vi "read.vi"(8 "error in (no error)":errorcluster, 11 "ValuePass in":refnum<class "RPCVariable.lvclass">) -> (0 "error out":errorcluster, 1 "Numeric":dbl, 2 "String":string, 3 "ValuePass out":refnum<class "RPCVariable.lvclass">)   [LabVIEW 2011, in "mbed_LVLibrary.lvlib" / "RPCVariable.lvclass"]
doc: "This VI will read the value of an RPCVariable on mbed. If the value is numeric it will be avalible on the numeric pin in number format, otherwise if it cannot be formatted to a number it will only be avalible as a string. When using this you need to be aware of the type of the variable attached on mbed."
uses:
  RPCVariable.lvclass
  RPCVariable.lvclass/RPCVariable.ctl
  Transport Mechanisms/mbed/mbed.lvclass
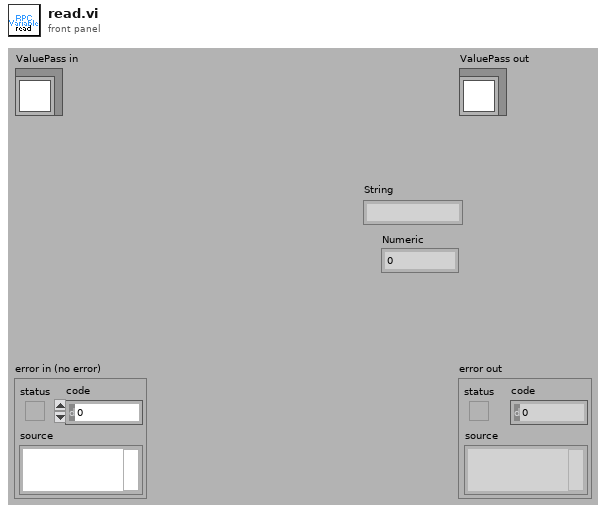
[diagram p1: front panel]
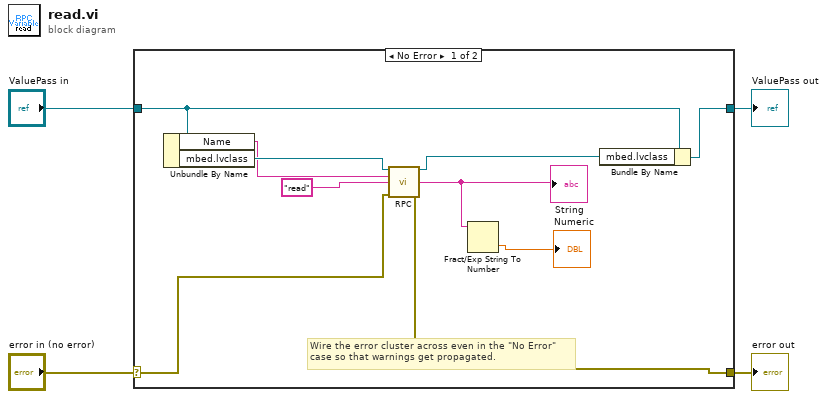
[diagram p0: block diagram]
diagram:
  n1 = case shown="No Error" "error in (no error)" {
    selector: "error in (no error)" -> [w8 w16]
    tunnel: [w7 w16] -> w3
    tunnel: [w13 w15] -> w1
    tunnel: "ValuePass in" -> [w14 w15]
    frame No Error {
      # "Wire the error cluster across even in the \"No Error\"\ncase so that warnings get propagated."
      n2 = Unbundle By Name(w14) -> ("Name"=w11:string, "mbed.lvclass"=w12:refnum<class "mbed.lvclass">)
      n3 = call-dynamic "RPC.vi"("mbed in"=w12, "Name"=w11, "method"="read", "error in (no error)"=w8) -> ("mbed out"=w10:refnum<class "mbed.lvclass">, "RPC Result"=w6:string, "error out"=w7:errorcluster)  [unwired: 9 in]
      "String" <- w6
      n4 = Fract/Exp String To Number(string=w6) -> (number=→"Numeric":dbl)  [unwired: 3 in, 1 out]
      n5 = Bundle By Name(cluster=w14, "mbed.lvclass"=w10) -> (w13:refnum<class "RPCVariable.lvclass">)
    }
    frame Error {
    }
  }
  "error out" <- w3
  "ValuePass out" <- w1
